vi "Teleop.vi"(10 "Match Info":T1={"Autonomous Elapsed Seconds"=0.0, "TeleOp Elapsed Seconds"=0.0, "Disabled Elapsed Seconds"=0.0, "Visited Autonomous"=FALSE, "Visited TeleOp"=FALSE, "Visited Disabled"=FALSE, "Autonomous Settings"={"Autonomous Style"=enum."Independent", "VI Refnum"=refnum}}, 11 "Call Context":T2) -> ()   [LabVIEW 2019]
doc: "This VI is called for each TeleOp packet received from the DS where the robot is not disabled. It is often used to read from the joysticks and update I/O or to update setpoints for timed control loops. It should complete and return within 20 milliseconds or it may miss DS packets."
uses:
  <vilib>/Rock Robotics/WPI/DriverStation/WPI_DriverStationDerivedRobotMode.ctl
  <vilib>/Rock Robotics/WPI/DriverStation/WPI_DriverStationMatch Info.ctl
  <vilib>/Rock Robotics/WPI/Utilities/WPI_GetSetVariantRefNum.vi
  Robot Global Data.vi
  <vilib>/Rock Robotics/Network Tables/NT Write Number.vi
  <vilib>/Rock Robotics/Network Tables/NT Write Numeric Array.vi
  <vilib>/Rock Robotics/Network Tables/NT Write Boolean Array.vi
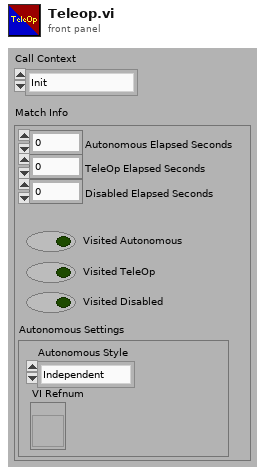
[diagram p1: front panel]
types:
  T1 = typedef "WPI_DriverStationMatch Info.ctl" = cluster{"Autonomous Elapsed Seconds":dbl, "TeleOp Elapsed Seconds":dbl, "Disabled Elapsed Seconds":dbl, "Visited Autonomous":bool, "Visited TeleOp":bool, "Visited Disabled":bool, "Autonomous Settings":cluster{"Autonomous Style":enum16{"Iterative", "Independent"}, "VI Refnum":refnum<vi>}}
  T2 = typedef "WPI_DriverStationDerivedRobotMode.ctl" = enum16{"Init", "Execute", "Stop"}
  T3 = typedef "WPI_JoystickDevRef.ctl" = cluster{"Device":T4}
  T4 = typedef "WPI_JoystickDeviceEnum.ctl" = enum16{"USB 0", "USB 1", "USB 2", "USB 3", "USB 4", "USB 5"}
  T5 = typedef "WPI_RobotDriveDevRef.ctl" = cluster{"DevStatus":errorcluster, "Motors[]":T6[], "Square Inputs":bool, "Max Output":dbl}
  T6 = typedef "WPI_MotorControlDeviceRef.ctl" = cluster{"DeviceStatus":errorcluster, "Type":T7, "PWM":cluster{"PWM Channel":T8, "DeadBand":T9}, "CAN":cluster{"Device Number":u8, "SetOutput VI Ref":variant, "GetOutput VI Ref":variant, "Enable VI Ref":variant, "Disable VI Ref":variant, "Data":variant}, "Invert":bool, "DIO PWM":cluster{"PWM \"Enable\" Channel":T8, "DIOChannel":T10, "PWM Rate":dbl}}
  T7 = typedef "WPI_MotorControlType.ctl" = enum16{"PWM", "CAN", "DIO PWM"}
  T8 = typedef "FPGA_DIOPWMChannel.ctl" = enum8{"PWM 0", "PWM 1", "PWM 2", "PWM 3", "PWM 4", "PWM 5", "PWM 6", "PWM 7", "PWM 8", "PWM 9", "PWM MXP 0", "PWM MXP 1", "PWM MXP 2", "PWM MXP 3", "PWM MXP 4", "PWM MXP 5", "PWM MXP 6", "PWM MXP 7", "PWM MXP 8", "PWM MXP 9", "Invalid"}
  T9 = typedef "WPI_PWMDeadband.ctl" = cluster{"Name":string, "maxPositivePwm":i32, "minPositivePwm":i32, "centerPwm":i32, "maxNegativePwm":i32, "minNegativePwm":i32, "angularRange":u16}
  T10 = typedef "FPGA_DIOChannel.ctl" = enum8{"DIO 0", "DIO 1", "DIO 2", "DIO 3", "DIO 4", "DIO 5", "DIO 6", "DIO 7", "DIO 8", "DIO 9", "DIO MXP 0", "DIO MXP 1", "DIO MXP 2", "DIO MXP 3", "DIO MXP 4", "DIO MXP 5", "DIO MXP 6", "DIO MXP 7", "DIO MXP 8", "DIO MXP 9", "DIO MXP 10", "DIO MXP 11", "DIO MXP 12", "DIO MXP 13", "DIO MXP 14", "DIO MXP 15", "SPI Port CS1", "SPI Port CS2", "SPI Port CS3", "SPI Port MISO", "SPI Port MOSI", "Invalid"}
  T11 = cluster{"JoystickDevRef":T3, "RobotDriveDevRef":T5}
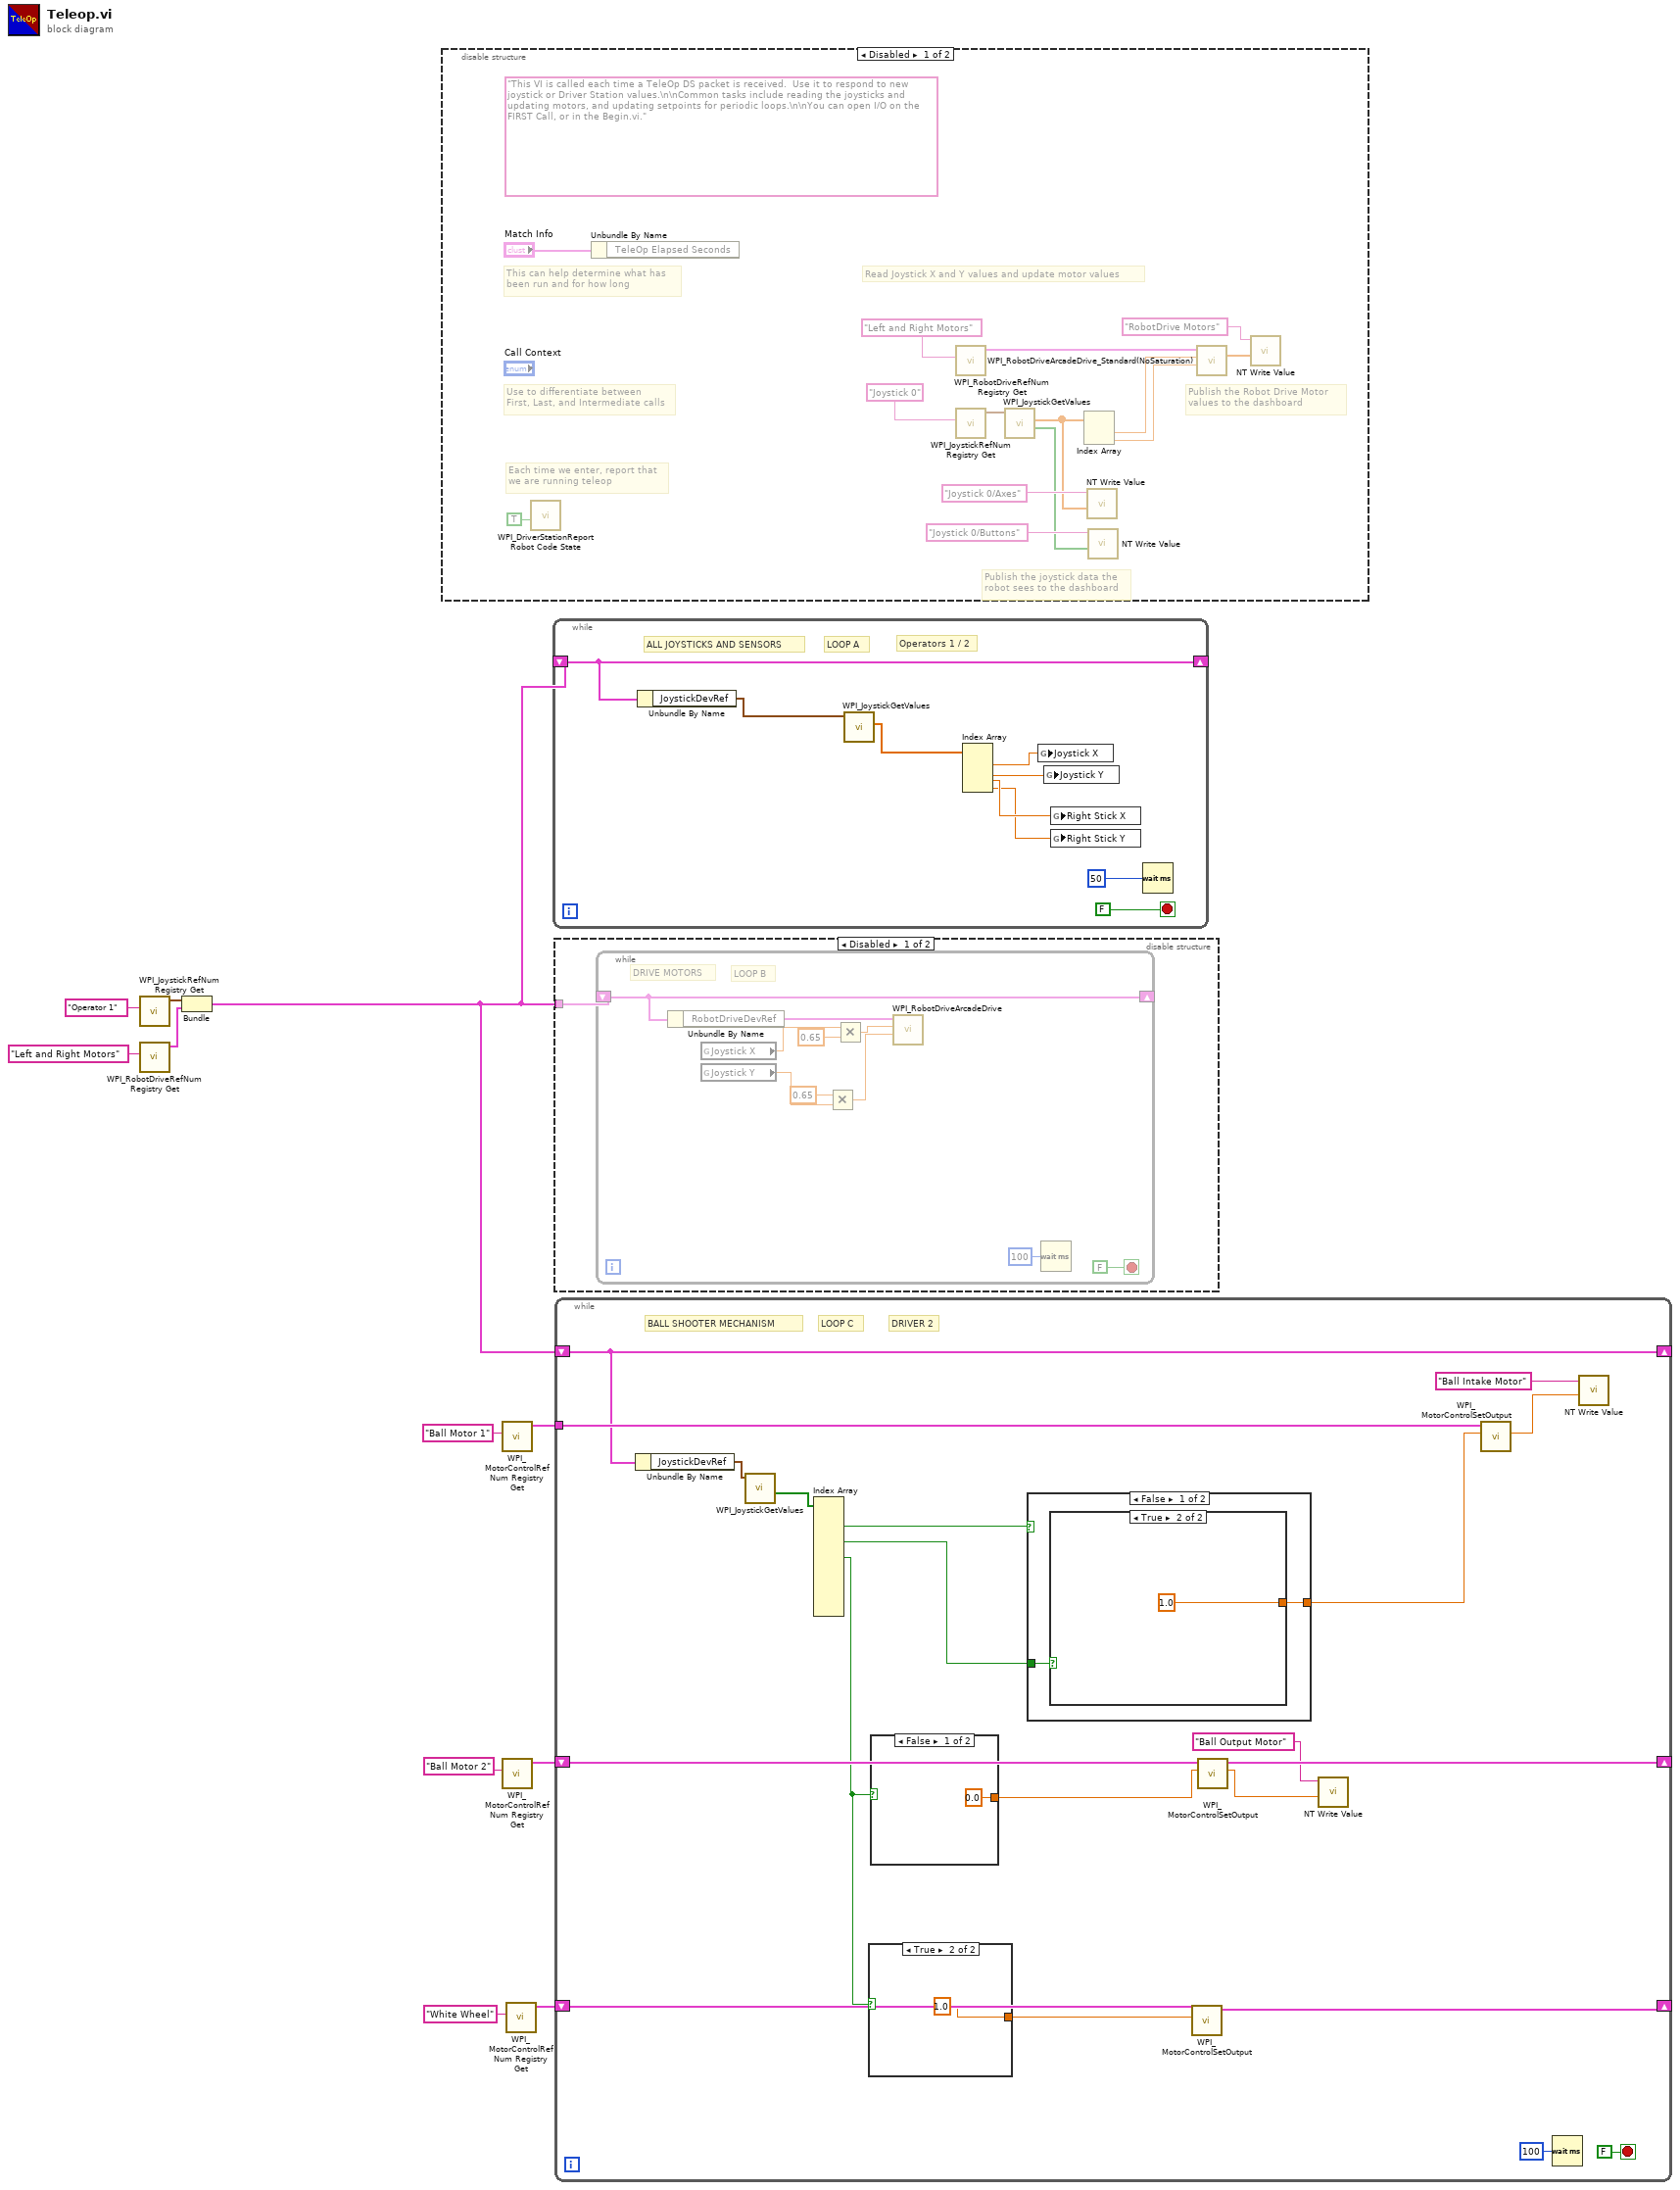
[diagram p0: block diagram]
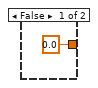
[diagram p4: hidden frame]
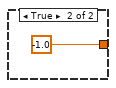
[diagram p5: hidden frame]
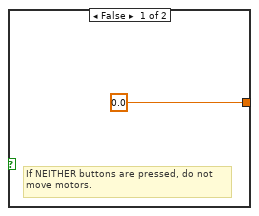
[diagram p6: hidden frame]
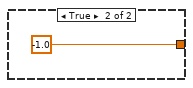
[diagram p7: hidden frame]
diagram:
  n1 = call <vilib>:"WPI_JoystickRefNum Registry Get.vi"("refnum name"="Operator 1") -> ("JoystickDevRef"=w9:T3)  [unwired: 1 in, 9 out]
  n2 = call <vilib>:"WPI_RobotDriveRefNum Registry Get.vi"("refnum name"="Left and Right Motors") -> ("RobotDriveDevRef"=w8:T5)  [unwired: 1 in, 9 out]
  n3 = Bundle("JoystickDevRef"=w9, "RobotDriveDevRef"=w8) -> (w1:T11)  [unwired: 1 out]
  n4 = disable-structure shown="Disabled" {
    frame Disabled {
      (unwired) "This VI is called each time a TeleOp DS packet is received.  Use it to respond to new joystick or Driver Station values.\n\nCommon tasks include reading the joysticks and updating motors, and updating setpoints for periodic loops.\n\nYou can open I/O on the FIRST Call, or in the Begin.vi."
      # "Publish the Robot Drive Motor\nvalues to the dashboard"
      # "Publish the joystick data the\nrobot sees to the dashboard"
      # "Each time we enter, report that\nwe are running teleop"
      # "Use to differentiate between\nFirst, Last, and Intermediate calls"
      # "This can help determine what has\nbeen run and for how long"
      # "Read Joystick X and Y values and update motor values"
      n5 = call <vilib>:"WPI_DriverStationReport Robot Code State.vi"("TeleOp"=TRUE ("Autonomous")) -> ()  [unwired: 10 in, 1 out]
      n6 = Unbundle By Name("Match Info") -> ()  [unwired: 1 out]
      n7 = call <vilib>:"WPI_RobotDriveRefNum Registry Get.vi"("refnum name"="Left and Right Motors") -> ("RobotDriveDevRef"=w23:T5)  [unwired: 1 in, 9 out]
      n8 = call <vilib>:"WPI_JoystickRefNum Registry Get.vi"("refnum name"="Joystick 0") -> ("JoystickDevRef"=w20:T3)  [unwired: 1 in, 9 out]
      n9 = call <vilib>:"WPI_JoystickGetValues.vi"("JoystickDevRef"=w20) -> ("Buttons"=w14:bool[], "Axes"=w15:dbl[])  [unwired: 6 in, 3 out]
      n10 = Index Array(array=w15) -> (element #1=w22:dbl, element #2=w18:dbl)  [unwired: 2 in]
      n11 = call-poly <vilib>:"NT Write Value.vi"("Numeric Array"=w15, "Name"="Joystick 0/Axes") -> ()  [unwired: 9 in, 1 out]
      n12 = call-poly <vilib>:"NT Write Value.vi"("Boolean Array"=w14, "Name"="Joystick 0/Buttons") -> ()  [unwired: 9 in, 1 out]
      n13 = call <vilib>:"WPI_RobotDriveArcadeDrive_Standard(NoSaturation).vi"("Y axis value"=w18, "X axis value"=w22, "RobotDriveDevRef"=w23) -> ("Motor Values"=w13:dbl[])  [unwired: 1 in, 7 out]
      n14 = call-poly <vilib>:"NT Write Value.vi"("Numeric Array"=w13, "Name"="RobotDrive Motors") -> ()  [unwired: 9 in, 1 out]
    }
    frame Enabled {
    }
  }
  n15 = call <vilib>:"WPI_MotorControlRefNum Registry Get.vi"("refnum name"="Ball Motor 1") -> ("MotorControlDevRef"=w6:T6)  [unwired: 9 in, 1 out]
  n16 = call <vilib>:"WPI_MotorControlRefNum Registry Get.vi"("refnum name"="Ball Motor 2") -> ("MotorControlDevRef"=w4:T6)  [unwired: 9 in, 1 out]
  n17 = call <vilib>:"WPI_MotorControlRefNum Registry Get.vi"("refnum name"="White Wheel") -> ("MotorControlDevRef"=w3:T6)  [unwired: 9 in, 1 out]
  n18 = while {
    shift-right: [w33] -> _
    shift-left: w1 -> [w33]
    stop <- FALSE stop-if-true
    # "Operators 1 / 2"
    # "LOOP A"
    # "ALL JOYSTICKS AND SENSORS"
    n19 = Unbundle By Name(w33) -> ("JoystickDevRef"=w32:T3)
    n20 = call <vilib>:"WPI_JoystickGetValues.vi"("JoystickDevRef"=w32) -> ("Axes"=w31:dbl[])  [unwired: 6 in, 4 out]
    n21 = Index Array(array=w31) -> (element #1=w29:dbl, element #2=w30:dbl, element #3=w27:dbl, element #4=w26:dbl)  [unwired: 4 in]
    n22 = global write "Robot Global Data.vi" "Joystick X"(w29) -> ()
    n23 = global write "Robot Global Data.vi" "Joystick Y"(w30) -> ()
    n24 = global write "Robot Global Data.vi" "Right Stick X"(w27) -> ()
    n25 = global write "Robot Global Data.vi" "Right Stick Y"(w26) -> ()
    n26 = Wait (ms)(milliseconds to wait=u32 50) -> ()  [unwired: 1 out]
  }
  n27 = disable-structure shown="Disabled" {
    disable-tunnel: w1 -> [w35 _]
    frame Disabled {
      n28 = while {
        shift-right: [w43] -> _
        shift-left: w35 -> [w43]
        stop <- FALSE stop-if-true
        # "DRIVE MOTORS"
        # "LOOP B"
        n29 = Unbundle By Name(w43) -> ("RobotDriveDevRef"=w42:T5)
        n30 = global read "Robot Global Data.vi" "Joystick X"() -> (w40:dbl)
        n31 = global read "Robot Global Data.vi" "Joystick Y"() -> (w41:dbl)
        n32 = Multiply(x=0.65, y=w41) -> (x*y=w37:dbl)
        n33 = Multiply(x=w40, y=0.65) -> (x*y=w36:dbl)
        n34 = call-poly <vilib>:"WPI_RobotDriveArcadeDrive.vi"("Y axis value"=w37, "X axis value"=w36, "RobotDriveDevRef"=w42) -> ()  [unwired: 6 in, 3 out]
        n35 = Wait (ms)(milliseconds to wait=u32 100) -> ()  [unwired: 1 out]
      }
    }
    frame Enabled {
    }
  }
  n36 = while {
    tunnel: w6 -> [w63]
    shift-right: [w59] -> _
    shift-left: w4 -> [w60]
    shift-right: [w54] -> _
    shift-left: w1 -> [w54]
    shift-right: [w49] -> _
    shift-left: w3 -> [w50]
    stop <- FALSE stop-if-true
    # "DRIVER 2"
    # "LOOP C"
    # "BALL SHOOTER MECHANISM"
    n37 = Unbundle By Name(w54) -> ("JoystickDevRef"=w53:T3)
    n38 = call <vilib>:"WPI_JoystickGetValues.vi"("JoystickDevRef"=w53) -> ("Buttons"=w61:bool[])  [unwired: 6 in, 4 out]
    n39 = Index Array(array=w61) -> (element #2=w52:bool, element #4=w51:bool, element #6=w46:bool)  [unwired: 13 in, 10 out]
    n40 = case shown="True" w46 {
      tunnel: [0.0 ("Output") 1.0 ("Output")] -> w47
      frame False {
      }
      frame True {
      }
    }
    n41 = case shown="False" w46 {
      tunnel: [0.0 ("Output") -1.0 ("Output")] -> w48
      frame False {
      }
      frame True {
      }
    }
    n42 = case shown="False" w52 {
      tunnel: [w71 -1.0 ("Output")] -> w62
      tunnel: w51 -> [w70 _]
      frame False {
        n43 = case shown="True" w70 {
          tunnel: [0.0 ("Output") 1.0 ("Output")] -> w71
          frame False {
            # "If NEITHER buttons are pressed, do not\nmove motors."
          }
          frame True {
          }
        }
      }
      frame True {
      }
    }
    n44 = call <vilib>:"WPI_MotorControlSetOutput.vi"("Output"=w47, "MotorControlDevRef"=w50) -> ("MotorControlDevRef"=w49:T6)  [unwired: 7 in, 2 out]
    n45 = call <vilib>:"WPI_MotorControlSetOutput.vi"("Output"=w48, "MotorControlDevRef"=w60) -> ("Motor Output"=w56:dbl, "MotorControlDevRef"=w59:T6)  [unwired: 7 in, 1 out]
    n46 = call-poly <vilib>:"NT Write Value.vi"("Numeric"=w56, "Name"="Ball Output Motor") -> ()  [unwired: 9 in, 1 out]
    n47 = call <vilib>:"WPI_MotorControlSetOutput.vi"("Output"=w62, "MotorControlDevRef"=w63) -> ("Motor Output"=w58:dbl)  [unwired: 7 in, 2 out]
    n48 = Wait (ms)(milliseconds to wait=u32 100) -> ()  [unwired: 1 out]
    n49 = call-poly <vilib>:"NT Write Value.vi"("Numeric"=w58, "Name"="Ball Intake Motor") -> ()  [unwired: 9 in, 1 out]
  }
